vi "TL_check_stability.vi"(3 "queue DAQ":refnum<queue>, 5 "queue CAMERA":refnum<queue>, 7 "queue ASI stage":refnum<queue>, 8 "error in":errorcluster, 10 "Data cluster":T1, 11 "queue piezo":refnum<queue>) -> (0 "error out":errorcluster)   [LabVIEW 2015]
uses:
  CONTROLS/Q_camera_element.ctl
  CONTROLS/Q_MCL_piezo_element.ctl
  CONTROLS/Q_DAQ_element.ctl
  CONTROLS/Q_ASI_stage_element.ctl
  GLOBAL/Global_MCL_piezo.vi
  GLOBAL/Global_ABORT.vi
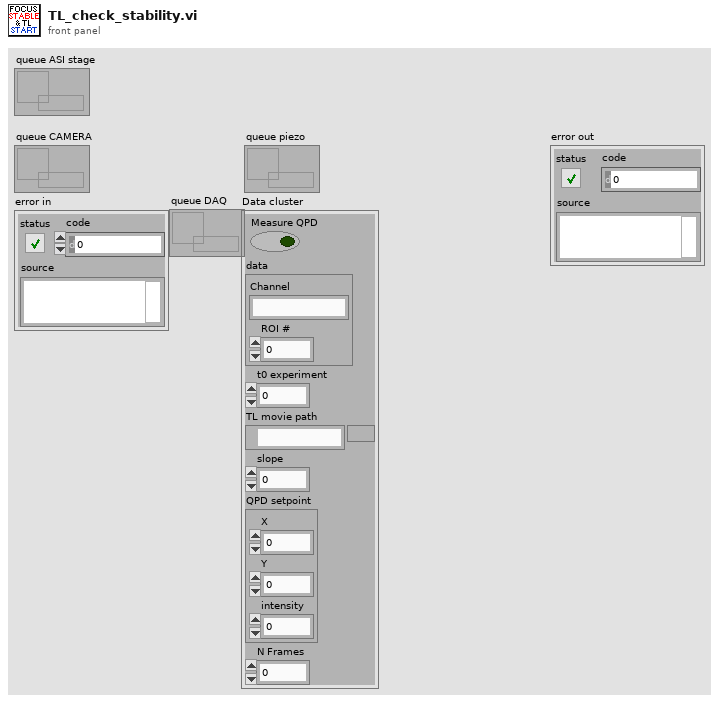
[diagram p1: front panel]
types:
  T1 = cluster{"Measure QPD":bool, "data":cluster{"Channel":string, "ROI #":i32}, "t0 experiment":dbl, "TL movie path":path, "slope":dbl, "QPD setpoint":cluster{"X":dbl, "Y":dbl, "intensity":dbl}, "N Frames":i32}
  T2 = typedef "Q_camera_element.ctl" = cluster{"variant":variant, "Instruction":enum16{"CAMERA_idle", "CAMERA_initialize", "CAMERA_error", "CAMERA_security_stop", "CAMERA_not_acquiring", "CAMERA_acquiring", "CAMERA_start_acquiring", "CAMERA_stop_acquiring", "CAMERA_change_exposure", "CAMERA_define_ROI", "CAMERA_cooler", "CAMERA_acquire_movie", "CAMERA_init_scan", "CAMERA_check_new_scan_image", "CAMERA_close_scan", "CAMERA_init_merFISH", "CAMERA_start_acquiring_merFISH", "CAMERA_close_scan_merFISH", "CAMERA_close_merFISH", "CAMERA_init_TL", "CAMERA_start_acquiring_TL", "CAMERA_stop_acquiring_TL", "CAMERA_close_TL", "CAMERA_STOP"}}
  T3 = typedef "Q_MCL_piezo_element.ctl" = cluster{"variant":variant, "Instruction":enum16{"Piezo_idle", "Piezo_initialize", "Piezo_error", "Piezo_security_stop", "Piezo_read_z", "Piezo_move_z", "Piezo_keyboard_move", "Piezo_close_autofocus_calibration_ramp", "Piezo_change_init_state", "Piezo_init_autofocus", "Piezo_init_autofocus_merFISH_TL", "Piezo_autofocus", "Piezo_autofocus_merFISH_TL", "Piezo_stop_autofocus", "Piezo_stop_autofocus_merFISH_TL", "Piezo_autofocus_lost", "Piezo_resume_autofocus_merFISH_TL", "Piezo_check_z_position_merFISH_TL", "Piezo_init_ramp", "Piezo_move_z_ramp", "Piezo_close_ramp", "Piezo_close_merFISH", "Piezo_init_TL", "Piezo_close_ramp_TL", "Piezo_close_TL", "Piezo_stop"}}
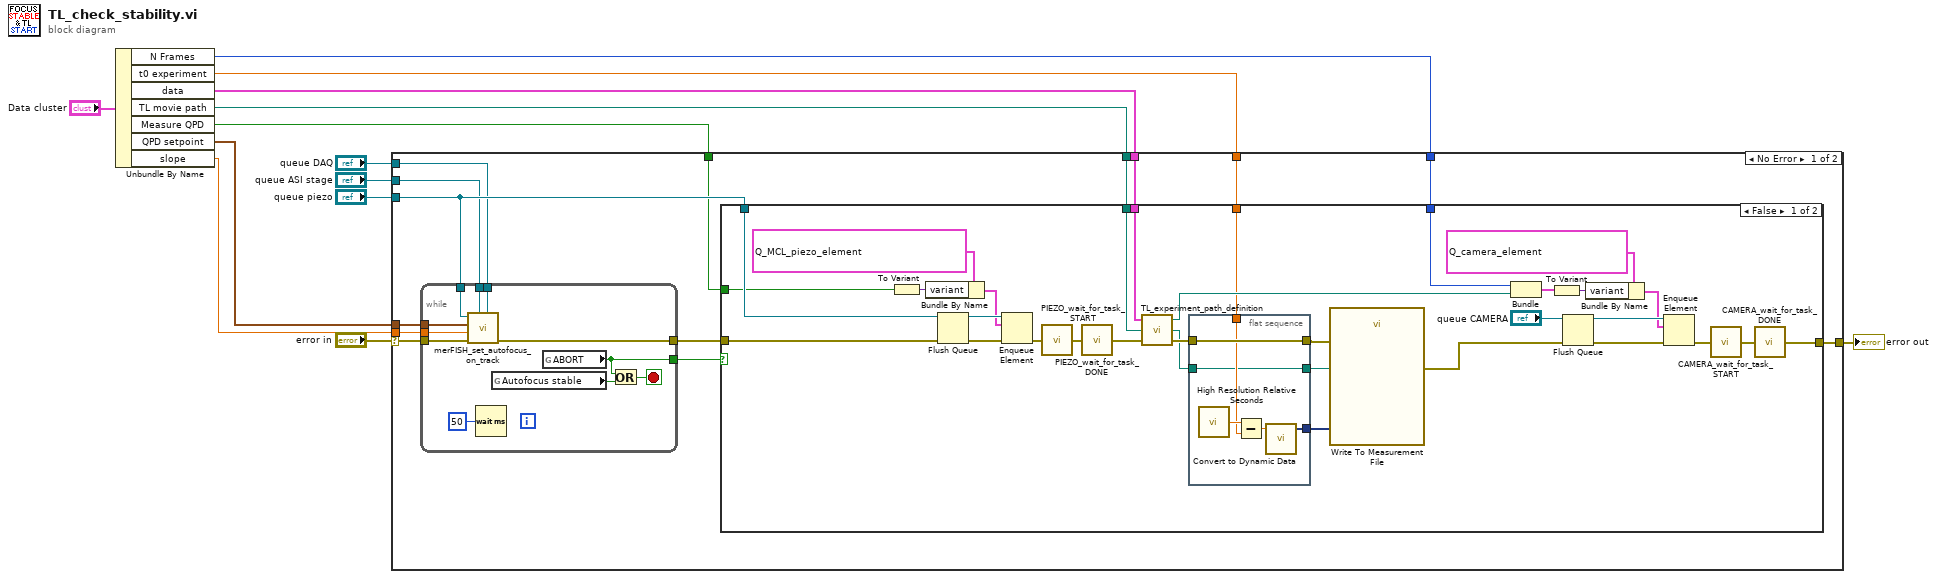
[diagram p0: block diagram]
diagram:
  n1 = Unbundle By Name("Data cluster") -> ("N Frames"=w2:i32, "t0 experiment"=w1:dbl, "data"=w4:cluster{"Channel":string, "ROI #":i32}, "TL movie path"=w5:path, "Measure QPD"=w6:bool, "QPD setpoint"=w7:cluster{"X":dbl, "Y":dbl, "intensity":dbl}, "slope"=w8:dbl)
  n2 = case shown="No Error" "error in" {
    selector: "error in" -> [w24 w78]
    tunnel: [w26 w78] -> w13
    tunnel: "queue piezo" -> [w23 _]
    tunnel: "queue DAQ" -> [w22 _]
    tunnel: w7 -> [w21 _]
    tunnel: "queue ASI stage" -> [w20 _]
    tunnel: w8 -> [w19 _]
    tunnel: w6 -> [w18 _]
    tunnel: w5 -> [w17 _]
    tunnel: w4 -> [w16 _]
    tunnel: w2 -> [w15 _]
    tunnel: w1 -> [w14 _]
    frame No Error {
      n3 = while {
        tunnel: w24 -> [w73]
        tunnel: [w72] -> w27
        tunnel: [w74] -> w25
        tunnel: w23 -> [w69]
        tunnel: w22 -> [w71]
        tunnel: w21 -> [w70]
        tunnel: w20 -> [w68]
        tunnel: w19 -> [w67]
        stop <- w75 stop-if-true
        n4 = call "merFISH_set_autofocus_on_track.vi"("queue DAQ"=w71, "queue ASI stage"=w68, "error in"=w73, "Slope"=w67, "QPD ref"=w70, "queue piezo"=w69) -> ("error out"=w72:errorcluster)  [unwired: 3 in]
        n5 = Wait (ms)(milliseconds to wait=u32 50) -> ()  [unwired: 1 out]
        n6 = global read "Global_MCL_piezo.vi" "Autofocus stable"() -> (w76:bool)
        n7 = global read "Global_ABORT.vi" "ABORT"() -> (w74:bool)
        n8 = Or(x=w74, y=w76) -> (x .or. y?=w75:bool)
      }
      n9 = case shown="False" w25 {
        tunnel: w27 -> [w50 w66]
        tunnel: [w49 w66] -> w26
        tunnel: w23 -> [w45 _]
        tunnel: w18 -> [w40 _]
        tunnel: w17 -> [w39 _]
        tunnel: w16 -> [w38 _]
        tunnel: w15 -> [w37 _]
        tunnel: w14 -> [w33 _]
        frame False {
          n10 = To Variant(anything=w40) -> (Variant=w47:variant)
          n11 = Bundle By Name(cluster=T3 {"variant"=variant, "Instruction"=enum."Piezo_stop_autofocus_merFISH_TL"} ("element"), "variant"=w47) -> (w46:T3)
          n12 = Flush Queue(queue=w45, error in (no error)=w50) -> (queue out=w51:refnum<queue>, error out=w52:errorcluster)  [unwired: 1 out]
          n13 = Enqueue Element(queue=w51, element=w46, error in (no error)=w52) -> (error out=w53:errorcluster)  [unwired: 1 in, 2 out]
          n14 = call "PIEZO_wait_for_task_START.vi"("error in"=w53) -> ("error out"=w54:errorcluster)
          n15 = call "PIEZO_wait_for_task_DONE.vi"("error in"=w54) -> ("error out"=w41:errorcluster)
          n16 = call "TL_experiment_path_definition.vi"("error in"=w41, "Path to the time lapse saving folder"=w39, "data"=w38) -> ("error out"=w34:errorcluster, "time file path"=w29:path, "movie path"=w36:path)
          n17 = flat-sequence {
            tunnel: w34 -> [w64]
            tunnel: w33 -> [w63]
            tunnel: [w64] -> w31
            tunnel: [w61] -> w32
            tunnel: [w60] -> w30
            tunnel: w29 -> [w60]
            frame #0 {
              n18 = call <vilib>:"High Resolution Relative Seconds.vi"() -> ("relative seconds"=w65:dbl)
              n19 = Subtract(x=w65, y=w63) -> (x-y=w62:dbl)
              n20 = call "Convert to Dynamic Data"("Double"=w62) -> ("Dynamic Data Type"=w61:dynamicdata)  [unwired: 3 in]
            }
          }
          n21 = call "Write To Measurement File"("Signals"=w32, "error in (no error)"=w31, "Filename"=w30) -> ("error out"=w28:errorcluster)  [unwired: 14 in, 2 out]
          n22 = Bundle("N Frames"=w37, "movie path"=w36) -> (w35:cluster{"N Frames":i32, "movie path":path})  [unwired: 1 in]
          n23 = To Variant(anything=w35) -> (Variant=w44:variant)
          n24 = Flush Queue(queue="queue CAMERA", error in (no error)=w28) -> (queue out=w57:refnum<queue>, error out=w58:errorcluster)  [unwired: 1 out]
          n25 = Bundle By Name(cluster=T2 {"variant"=variant, "Instruction"=enum."CAMERA_start_acquiring_TL"} ("Q_ANDOR_element"), "variant"=w44) -> (w43:T2)
          n26 = Enqueue Element(queue=w57, element=w43, error in (no error)=w58) -> (error out=w56:errorcluster)  [unwired: 1 in, 2 out]
          n27 = call "CAMERA_wait_for_task_START.vi"("error in"=w56) -> ("error out"=w55:errorcluster)
          n28 = call "CAMERA_wait_for_task_DONE.vi"("error in"=w55) -> ("error out"=w49:errorcluster)
        }
        frame True {
        }
      }
    }
    frame Error {
    }
  }
  "error out" <- w13
